vi "Setpoint.vi"(0 "GPIB ADDRESS":string, 2 "SET POINT":dbl(slide) scale=0.0..200.0 scale format="%.1f", 3 "?":bool) -> (1 "SET POINT VALUE":string)   [LabVIEW 2024]
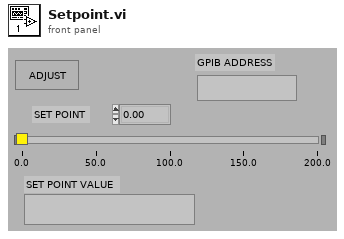
[diagram p1: front panel]
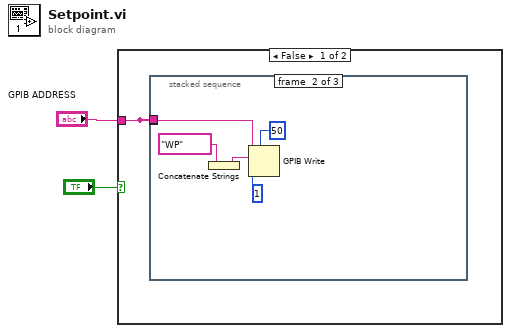
[diagram p0: block diagram]
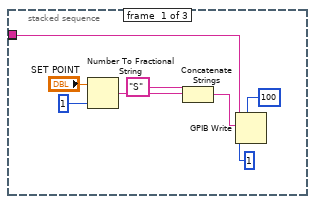
[diagram p2: hidden frame]
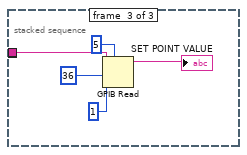
[diagram p3: hidden frame]
diagram:
  n1 = case shown="False" "?" {
    tunnel: "GPIB ADDRESS" -> [w3 _]
    frame False {
      n2 = stacked-sequence {
        tunnel: w3 -> [w5 w14 _]
        tunnel: w3 -> [_ _ w17]
        frame #0 {
          n3 = Number To Fractional String(number="SET POINT", precision (6)=1) -> (F-format string=w4:string)  [unwired: 2 in]
          n4 = Concatenate Strings("S", w4) -> (w6:string)
          n5 = GPIB Write(0:w5, 1:w6, 2:1, 4:100) -> ()  [unwired: 1 in, 2 out]
        }
        frame #1 {
          n6 = Concatenate Strings("WP") -> (w12:string)
          n7 = GPIB Write(0:w14, 1:w12, 2:1, 4:50) -> ()  [unwired: 1 in, 2 out]
        }
        frame #2 {
          n8 = GPIB Read(0:w17, 1:36, 2:1, 4:5) -> (5:→"SET POINT VALUE":string)  [unwired: 1 in, 2 out]
        }
      }
    }
    frame True {
    }
  }
